vi "SOUR_POW_CORR_COLL_SAVE.vi"(0 "VISA IN":refnum<visa-resource-name>, 1 "Port number":i32, 5 "error in":errorcluster, 7 "Channel":i32) -> (14 "VISA Out":refnum<visa-resource-name>, 19 "error out":errorcluster)   [LabVIEW 2018, in "PNA-X.lvlib"]
doc: "SOURce<cnum>:POWer<port>:CORRection:COLLect:SAVE [<RREC>] \n(Write-only) Applies the array of correction values after a source power calibration sweep has \ncompleted. The source power correction will then be active on the specified source port for channel \n<cnum>. This command does NOT save the correction values. To save correction values, save an \ninstrument / calibration state (*.cst file) after performing a source power cal. \nParameters \n<cnum> Any existing channel number. If unspecified, value is set to 1 \n<port> Port number to correct for source power. If unspecified, value is set to 1. \n<RREC> Optional argument. \nRRECeiver In addition to a source Power Cal, perform a calibration of the \nreference receiver used in the measurement. ONLY the Reference Receiver \ncalibration is then saved to a Cal Set or Cal Register as specified by the current \nsetting of SENS:CORR:PREF:CSET:SAVE. \nExamples SOUR:POW:CORR:COLL:SAVE \nsource1:power2:correction:collect:save rreceiver \nQuery Syntax Not Applicable \nDefault Not Applicable"
uses:
  PNA-X.lvlib
panel:
  out "resulting string":string
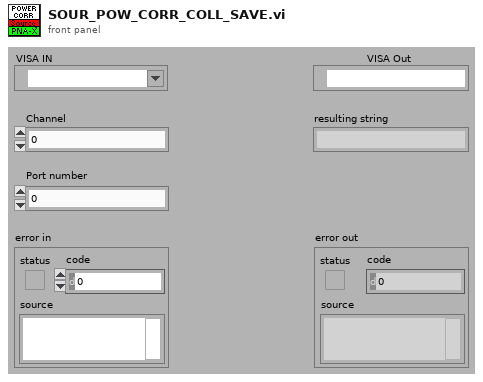
[diagram p1: front panel]
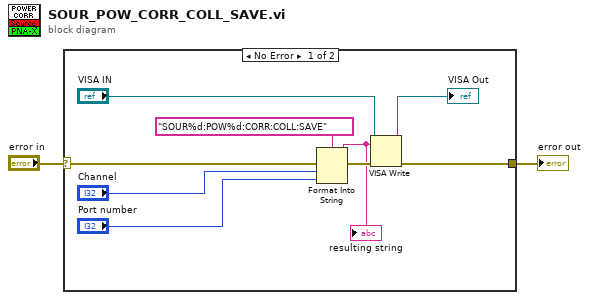
[diagram p0: block diagram]
diagram:
  n1 = case shown="No Error" "error in" {
    selector: "error in" -> [w11 w12]
    tunnel: [w6 w12] -> w1
    frame No Error {
      n2 = Format Into String(format string="SOUR%d:POW%d:CORR:COLL:SAVE" ("Cmdline"), error in=w11, "Channel", "Port number") -> (resulting string=w9:string, error out=w10:errorcluster)  [unwired: 1 in]
      "resulting string" <- w9
      n3 = VISA Write(VISA resource name="VISA IN", write buffer=w9, error in (no error)=w10) -> (VISA resource name out=→"VISA Out":refnum<visa-resource-name>, error out=w6:errorcluster)  [unwired: 1 out]
    }
    frame Error {
    }
  }
  "error out" <- w1
